vi "serialization tests.vi"() -> (0 "serialization error":errorcluster, 1 "validation error":errorcluster, 2 "modules equal":bool, 3 "channels equal":bool)   [LabVIEW 2013, in "alarms module tests.lvlib"]
uses:
  alarms module tests.lvlib
  module/configuration/alarms module configuration.lvclass
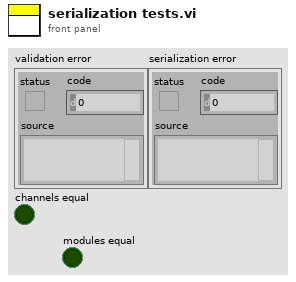
[diagram p1: front panel]
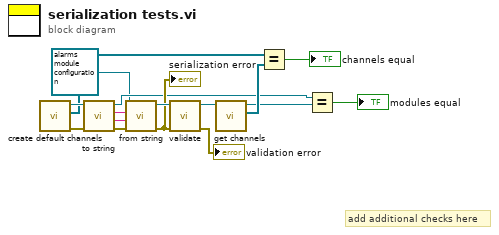
[diagram p0: block diagram]
diagram:
  # "add additional checks here"
  n1 = call "create default channels.vi"() -> ("error out"=w6:errorcluster, "channels"=w5:refnum<class "TBM channel.lvclass">[], "module"=w7:refnum<class "alarms module configuration.lvclass">)  [unwired: 7 in, 2 out]
  n2 = call-dynamic "to string.vi"("error in"=w6, "alarms module configuration in"=w7) -> ("error out"=w16:errorcluster, "data"=w15:string, "version"=w14:string, "alarms module configuration out"=w2:refnum<class "alarms module configuration.lvclass">)  [unwired: 6 in]
  n3 = call-dynamic "from string.vi"("error in"=w16, "data"=w15, "version"=w14, "alarms module configuration in"=refnum<class "alarms module configuration.lvclass"> refnum ("tag bus configurable plugin module configuration")) -> ("error out"=w11:errorcluster, "alarms module configuration out"=w13:refnum<class "alarms module configuration.lvclass">)  [unwired: 6 in]
  "serialization error" <- w11
  n4 = call-dynamic "validate.vi"("error in"=w11, "alarms module configuration in"=w13) -> ("error out"=→"validation error":errorcluster, "alarms module configuration out"=w9:refnum<class "alarms module configuration.lvclass">)  [unwired: 8 in]
  n5 = call-dynamic "get channels.vi"("alarms module configuration in"=w9) -> ("channels"=w8:refnum<class "TBM channel.lvclass">[], "alarms module configuration out"=w3:refnum<class "alarms module configuration.lvclass">)  [unwired: 9 in]
  n6 = Equal?(x=w5, y=w8) -> (x = y?=→"channels equal":bool)
  n7 = Equal?(x=w2, y=w3) -> (x = y?=→"modules equal":bool)
